vi "Begin.vi"(8 "error in":errorcluster) -> (0 "error out":errorcluster)   [LabVIEW 2015]
doc: "Called before other user functions, this VI is expected to open initial I/O refnums, load in file data, and do all program initialization. Notice that the <B>error out</B> terminal is simply used for data flow. Wiring it to other structures or subVIs ensures that this VI runs first."
uses:
  <vilib>/Rock Robotics/SystemInterfaces/DIO/FPGA_DIOPWMChannel.ctl
  Robot Global Data.vi
  <vilib>/Rock Robotics/WPI/DriverStation/WPI_DriverStationRobotMode2.ctl
  <vilib>/Rock Robotics/WPI/Joystick/WPI_JoystickDeviceEnum.ctl
  <vilib>/Rock Robotics/Network Tables/NT Write String Array.vi
  <vilib>/Rock Robotics/WPI/MotorControl/WPI_MotorControlOpen Talon.vi
  <vilib>/Rock Robotics/WPI/MotorControl/WPI_MotorControlOpen Jaguar.vi
  <vilib>/Rock Robotics/WPI/Ultrasonic/WPI_SonarMB1010DigitalOpen.vi
  <vilib>/Rock Robotics/WPI/Ultrasonic/WPI_SonarMB1010DigRefNum Registry Set.vi
  <vilib>/Rock Robotics/WPI/Accelerometer/WPI_AccelerometerADXL362_SPI_Open.vi
  <vilib>/Rock Robotics/SystemInterfaces/spilib/spi_bus.ctl
  <vilib>/Rock Robotics/WPI/Accelerometer/ADXL362 Range.ctl
  <vilib>/Rock Robotics/WPI/Accelerometer/WPI_AccelerometerADXL345 Axes.ctl
panel:
  in  "ADXL345 Axes 2":T1={"X-Axis"=TRUE, "Y-Axis"=FALSE, "Z-Axis"=FALSE}
  in  "Accel Range 2":T2 items=["+/- 2 g", "+/- 4 g", "+/- 8 g"]
  in  "SPI Bus 2":T3=enum."SPI On-Board, CS1"
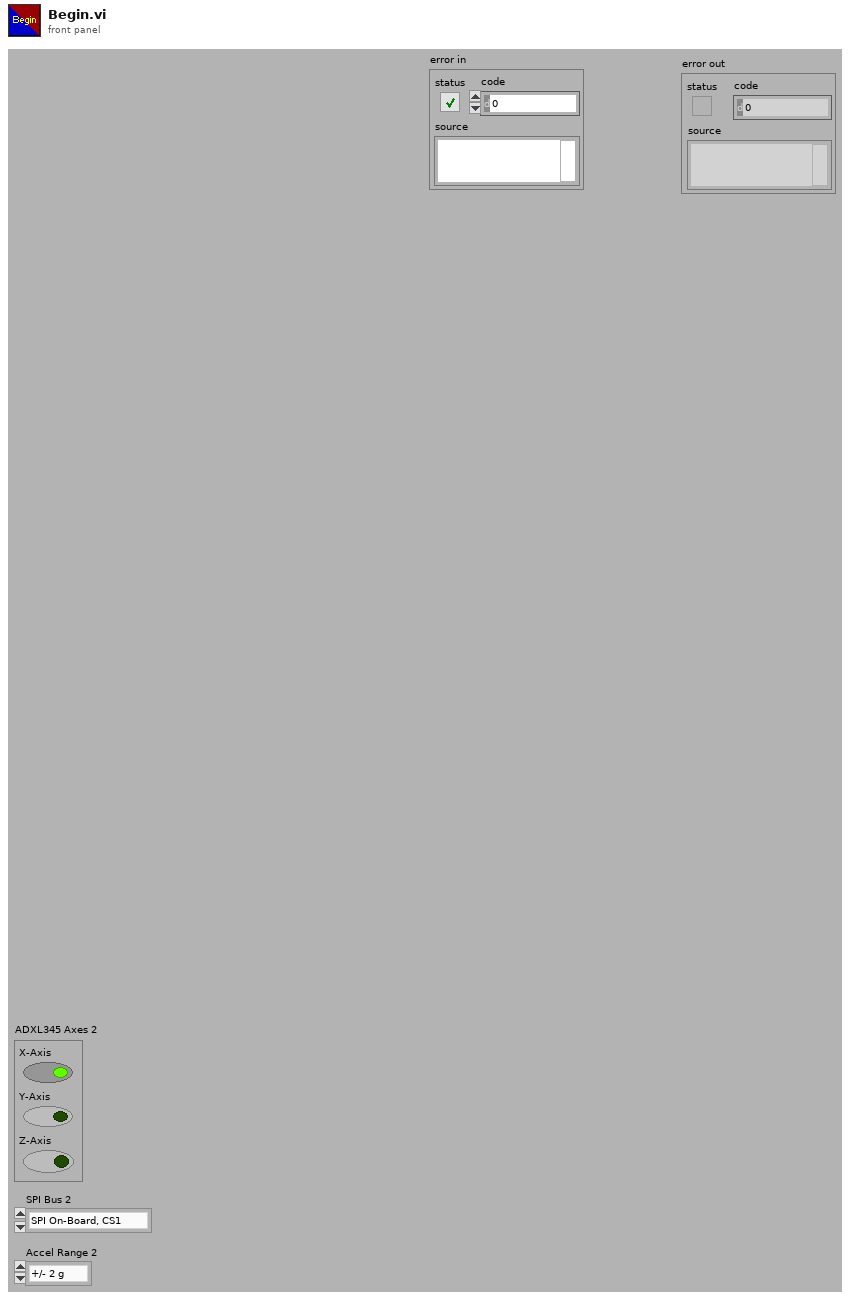
[diagram p1: front panel]
types:
  T1 = typedef "WPI_AccelerometerADXL345 Axes.ctl" = cluster{"X-Axis":bool, "Y-Axis":bool, "Z-Axis":bool}
  T2 = typedef "ADXL362 Range.ctl" = u8
  T3 = typedef "spi_bus.ctl" = enum16{"SPI On-Board, CS0", "SPI On-Board, CS1", "SPI On-Board, CS2", "SPI On-Board, CS3", "SPI MXP", "Invalid"}
  T4 = typedef "FPGA_DIOPWMChannel.ctl" = enum8{"PWM 0", "PWM 1", "PWM 2", "PWM 3", "PWM 4", "PWM 5", "PWM 6", "PWM 7", "PWM 8", "PWM 9", "PWM MXP 0", "PWM MXP 1", "PWM MXP 2", "PWM MXP 3", "PWM MXP 4", "PWM MXP 5", "PWM MXP 6", "PWM MXP 7", "PWM MXP 8", "PWM MXP 9", "Invalid"}
  T5 = typedef "WPI_JoystickDeviceEnum.ctl" = enum16{"USB 0", "USB 1", "USB 2", "USB 3", "USB 4", "USB 5"}
  T6 = typedef "WPI_DriverStationRobotMode2.ctl" = enum16{"Autonomous Disabled", "Autonomous Enabled", "Teleop Disabled", "Teleop Enabled", "Disconnected", "Finish", "Test Disabled", "Test Enabled", "Emergency Stopped"}
  T7 = typedef "WPI_AccelerometerDevRef.ctl" = cluster{"DevStatus":errorcluster, "Scaling":T8, "Analog Channels":T9, "I2C Bus":T11, "SPI Bus":T3, "Accel Range":T12, "ADXL Axes":T1, "Handle":i32, "Device Address":u8, "Accel Type":enum16{"Analog", "ADXL345 I2C", "ADXL345 SPI", "Internal", "ADXL362 SPI"}}
  T8 = typedef "WPI_AccelerometerScaling.ctl" = cluster{"Gain (VoltsPerG)":dbl, "Center Voltage":dbl}
  T9 = typedef "WPI_AccelerometerAnalogChannels.ctl" = cluster{"X-Axis":T10, "Y-Axis":T10, "Z-Axis":T10}
  T10 = typedef "FPGA_AIChannel.ctl" = enum8{"AI 0", "AI 1", "AI 2", "AI 3", "AI MXP 0", "AI MXP 1", "AI MXP 2", "AI MXP 3", "Invalid"}
  T11 = typedef "i2c_bus.ctl" = enum16{"I2C On-Board", "I2C MXP", "Invalid"}
  T12 = typedef "ADXL345 Range.ctl" = u8
  T13 = typedef "WPI_SonarMB1010DigitalDeviceRef.ctl" = cluster{"CounterDevRef":T14, "Scaling factor (s/in)":dbl}
  T14 = typedef "WPI_CounterDevRef.ctl" = cluster{"DevStatus":errorcluster, "CntIndex":T15}
  T15 = typedef "FPGA_CounterCtrSystemIndex.ctl" = enum8{"Ctr 0", "Ctr 1", "Ctr 2", "Ctr 3", "Ctr 4", "Ctr 5", "Ctr 6", "Ctr 7", "Invalid"}
  T16 = typedef "WPI_ServoDeviceRef.ctl" = cluster{"DeviceStatus":errorcluster, "PWM Channel":T4, "DeadBand":T17}
  T17 = typedef "WPI_PWMDeadband.ctl" = cluster{"Name":string, "maxPositivePwm":i32, "minPositivePwm":i32, "centerPwm":i32, "maxNegativePwm":i32, "minNegativePwm":i32, "angularRange":u16}
  T18 = typedef "WPI_JoystickDevRef.ctl" = cluster{"Device":T5}
  T19 = typedef "WPI_MotorControlDeviceRef.ctl" = cluster{"DeviceStatus":errorcluster, "Type":T20, "PWM":cluster{"PWM Channel":T4, "DeadBand":T17}, "CAN":cluster{"Device Number":u8, "Control Mode":T21, "Semaphore":T22, "Max Vout":dbl, "TalonSRX Control Mode":T23}, "Invert":bool}
  T20 = typedef "WPI_MotorControlType.ctl" = enum16{"PWM", "CAN", "CANTalonSRX"}
  T21 = typedef "WPI_CANJaguar_ControlMode.ctl" = enum8{"Percent VBus", "Current", "Speed", "Position", "Voltage"}
  T22 = typedef "Semaphore RefNum" = refnum<k1>
  T23 = typedef "WPI_CANTalonSRX_APIControlMode.ctl" = enum8{"Percent VBus", "Speed", "Position", "Slave", "Unchanged / Invalid", "Voltage Compensation", "Current", "Motion Profile"}
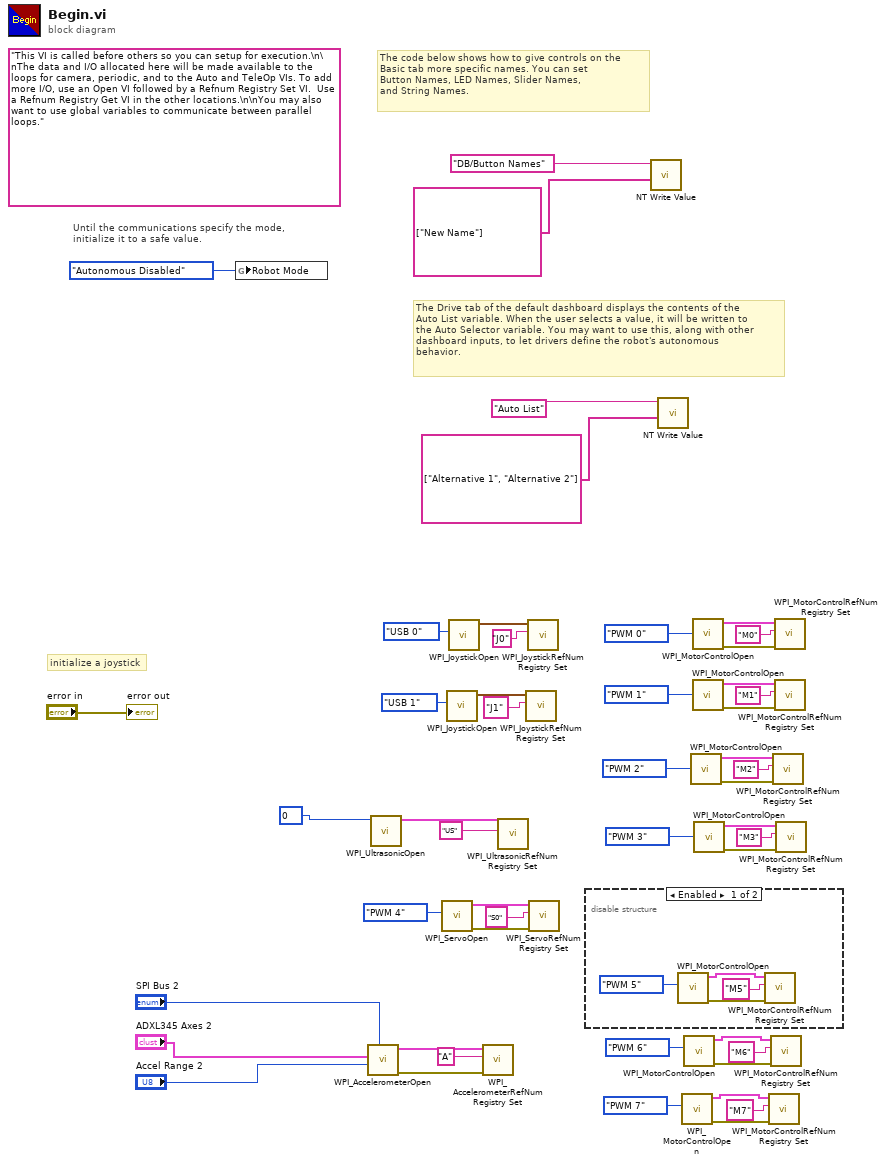
[diagram p0: block diagram]
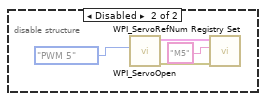
[diagram p2: hidden frame]
diagram:
  w4 = u16 0 items=[""]
  (unwired) "This VI is called before others so you can setup for execution.\n\nThe data and I/O allocated here will be made available to the loops for camera, periodic, and to the Auto and TeleOp VIs. To add more I/O, use an Open VI followed by a Refnum Registry Set VI.  Use a Refnum Registry Get VI in the other locations.\n\nYou may also want to use global variables to communicate between parallel loops."
  # "The Drive tab of the default dashboard displays the contents of the\nAuto List variable. When the user selects a value, it will be written to\nthe Auto Selector variable. You may want to use this, along with other\ndashboard inputs, to let drivers define the robot's autonomous\nbehavior."
  # "The code below shows how to give controls on the\nBasic tab more specific names. You can set\nButton Names, LED Names, Slider Names,\nand String Names."
  # "initialize a joystick"
  # "Until the communications specify the mode,\ninitialize it to a safe value."
  n1 = global write "Robot Global Data.vi" "Robot Mode"(WPI_DriverStationRobotMode2."Autonomous Disabled" ("Robot Mode")) -> ()
  n2 = call-poly <vilib>:"WPI_AccelerometerOpen.vi"("SPI Bus"="SPI Bus 2", "Accel Range"="Accel Range 2", "ADXL345 Axes"="ADXL345 Axes 2") -> ("error out"=w17:errorcluster, "AccelerometerDevRef"=w16:T7)  [unwired: 7 in]
  n3 = call-poly <vilib>:"WPI_UltrasonicOpen.vi"("DIO Channel"=w4) -> ("SonarMB1010DigitalDevRef"=w6:T13)  [unwired: 9 in, 1 out]
  n4 = call <vilib>:"WPI_ServoOpen.vi"("PWM Channel"=FPGA_DIOPWMChannel."PWM 4") -> ("error out"=w21:errorcluster, "ServoDeviceRef"=w20:T16)  [unwired: 9 in]
  n5 = call <vilib>:"WPI_JoystickOpen.vi"("JoystickDevice"=WPI_JoystickDeviceEnum."USB 1") -> ("JoystickDevRef"=w39:T18)  [unwired: 10 in]
  n6 = call <vilib>:"WPI_JoystickOpen.vi"("JoystickDevice"=WPI_JoystickDeviceEnum."USB 0") -> ("JoystickDevRef"=w47:T18)  [unwired: 10 in]
  n7 = call <vilib>:"WPI_AccelerometerRefNum Registry Set.vi"("error in (no error)"=w17, "refnum name"="A", "AccelerometerDevRef"=w16) -> ()  [unwired: 7 in, 2 out]
  n8 = call-poly <vilib>:"WPI_UltrasonicRefNum Registry Set.vi"("refnum name"="US", "SonarMB1010DigitalDevRef"=w6) -> ()  [unwired: 8 in, 2 out]
  n9 = call <vilib>:"WPI_JoystickRefNum Registry Set.vi"("refnum name"="J1", "JoystickDevRef"=w39) -> ()  [unwired: 8 in, 2 out]
  n10 = call <vilib>:"WPI_JoystickRefNum Registry Set.vi"("refnum name"="J0", "JoystickDevRef"=w47) -> ()  [unwired: 8 in, 2 out]
  n11 = call <vilib>:"WPI_ServoRefNum Registry Set.vi"("error in (no error)"=w21, "refnum name"="S0", "ServoDeviceRef"=w20) -> ()  [unwired: 7 in, 2 out]
  n12 = disable-structure shown="Enabled" {
    frame Enabled {
      n13 = call-poly <vilib>:"WPI_MotorControlOpen.vi"("PWM Channel"=FPGA_DIOPWMChannel."PWM 5") -> ("error out"=w53:errorcluster, "MotorControlDeviceRef"=w50:T19)  [unwired: 9 in]
      n14 = call <vilib>:"WPI_MotorControlRefNum Registry Set.vi"("error in (no error)"=w53, "refnum name"="M5", "MotorControlDevRef"=w50) -> ()  [unwired: 7 in, 2 out]
    }
    frame Disabled {
      n15 = call <vilib>:"WPI_ServoOpen.vi"("PWM Channel"=FPGA_DIOPWMChannel."PWM 5") -> ("error out"=w57:errorcluster, "ServoDeviceRef"=w56:T16)  [unwired: 9 in]
      n16 = call <vilib>:"WPI_ServoRefNum Registry Set.vi"("error in (no error)"=w57, "refnum name"="M5", "ServoDeviceRef"=w56) -> ()  [unwired: 7 in, 2 out]
    }
  }
  n17 = call-poly <vilib>:"NT Write Value.vi"("String Array"=string[] ["New Name"], "Name"="DB/Button Names") -> ()  [unwired: 9 in, 1 out]
  n18 = call-poly <vilib>:"NT Write Value.vi"("String Array"=string[] ["Alternative 1", "Alternative 2"], "Name"="Auto List") -> ()  [unwired: 9 in, 1 out]
  n19 = call-poly <vilib>:"WPI_MotorControlOpen.vi"("PWM Channel"=FPGA_DIOPWMChannel."PWM 7") -> ("error out"=w14:errorcluster, "MotorControlDeviceRef"=w11:T19)  [unwired: 9 in]
  n20 = call-poly <vilib>:"WPI_MotorControlOpen.vi"("PWM Channel"=FPGA_DIOPWMChannel."PWM 6") -> ("error out"=w10:errorcluster, "MotorControlDeviceRef"=w7:T19)  [unwired: 9 in]
  n21 = call-poly <vilib>:"WPI_MotorControlOpen.vi"("PWM Channel"=FPGA_DIOPWMChannel."PWM 2") -> ("error out"=w28:errorcluster, "MotorControlDeviceRef"=w27:T19)  [unwired: 9 in]
  n22 = call-poly <vilib>:"WPI_MotorControlOpen.vi"("PWM Channel"=FPGA_DIOPWMChannel."PWM 0") -> ("error out"=w36:errorcluster, "MotorControlDeviceRef"=w35:T19)  [unwired: 9 in]
  n23 = call-poly <vilib>:"WPI_MotorControlOpen.vi"("PWM Channel"=FPGA_DIOPWMChannel."PWM 1") -> ("error out"=w32:errorcluster, "MotorControlDeviceRef"=w31:T19)  [unwired: 9 in]
  n24 = call-poly <vilib>:"WPI_MotorControlOpen.vi"("PWM Channel"=FPGA_DIOPWMChannel."PWM 3") -> ("error out"=w24:errorcluster, "MotorControlDeviceRef"=w23:T19)  [unwired: 9 in]
  n25 = call <vilib>:"WPI_MotorControlRefNum Registry Set.vi"("error in (no error)"=w14, "refnum name"="M7", "MotorControlDevRef"=w11) -> ()  [unwired: 7 in, 2 out]
  n26 = call <vilib>:"WPI_MotorControlRefNum Registry Set.vi"("error in (no error)"=w10, "refnum name"="M6", "MotorControlDevRef"=w7) -> ()  [unwired: 7 in, 2 out]
  n27 = call <vilib>:"WPI_MotorControlRefNum Registry Set.vi"("error in (no error)"=w28, "refnum name"="M2", "MotorControlDevRef"=w27) -> ()  [unwired: 7 in, 2 out]
  n28 = call <vilib>:"WPI_MotorControlRefNum Registry Set.vi"("error in (no error)"=w36, "refnum name"="M0", "MotorControlDevRef"=w35) -> ()  [unwired: 7 in, 2 out]
  n29 = call <vilib>:"WPI_MotorControlRefNum Registry Set.vi"("error in (no error)"=w32, "refnum name"="M1", "MotorControlDevRef"=w31) -> ()  [unwired: 7 in, 2 out]
  n30 = call <vilib>:"WPI_MotorControlRefNum Registry Set.vi"("error in (no error)"=w24, "refnum name"="M3", "MotorControlDevRef"=w23) -> ()  [unwired: 7 in, 2 out]
  "error out" <- "error in"
